vi "My_DHT11_Labview1_Gweb.vi"() -> ()   [LabVIEW 2024]
uses:
  <vilib>/Instr/_visa.llb/VISA Configure Serial Port (Instr).vi
  GlobalHum1.vi
  GlobalFan2.vi
  GlobalTemp1.vi
  GlobalFan1.vi
panel:
  in  "Tab Control 2":enum32{"Hum Chart", "Hum Gauge"}(tab)
  out "Waveform Chart 2":dbl(graph)
  out "Gauge 2":dbl(knob) scale=0.0..100.0 scale format="%%%#_g"
  in  "Tab Control":enum32{"Temp Chart", "Temp Gauge"}(tab)
  out "Waveform Chart":dbl(graph)
  out "Gauge":dbl(knob) scale=0.0..50.0
  out "Fan LED 2":bool
  out "Fan LED":bool
  in  "Fan":bool
  out "Humidity":dbl(slide) scale=0.0..100.0 scale format="%%%d"
  out "Temperature":dbl(slide) scale=0.0..100.0
  in  "?":bool
  in  "VISA Arduino Uno":refnum<visa-resource-name>
  in  "Fan2":bool
  # "Environmental Control System for Greenhouses\n\nMonitoring System"
  # "House No. 1"
  # "C"
  # "%"
  # "Eng. Yahia Gaddal\ngaddal18@gmail.com"
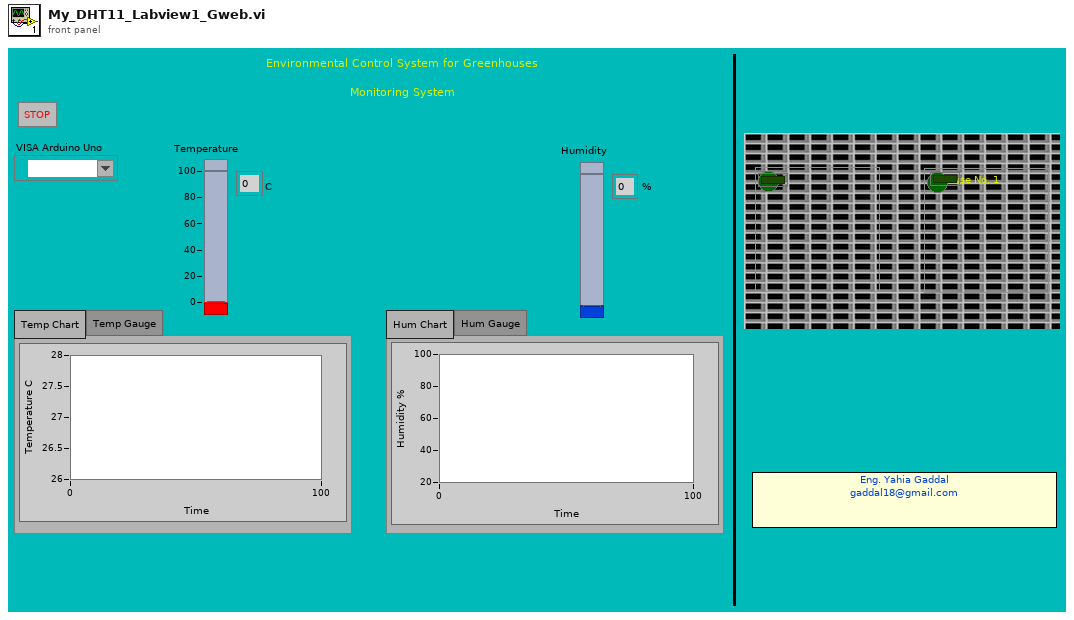
[diagram p1: front panel]
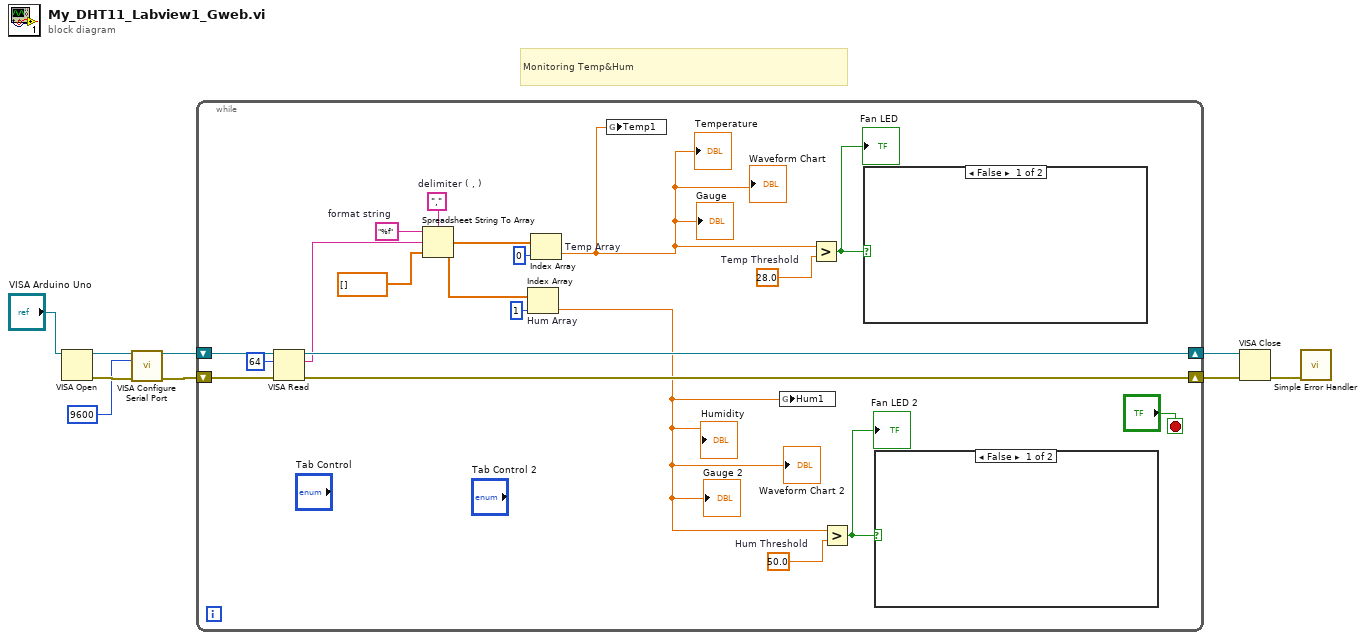
[diagram p0: block diagram]
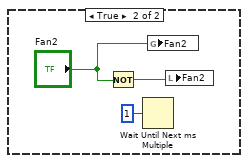
[diagram p2: hidden frame]
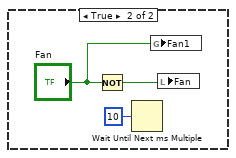
[diagram p3: hidden frame]
diagram:
  # "Monitoring Temp&Hum"
  n1 = VISA Open(VISA resource name="VISA Arduino Uno") -> (VISA resource name=w9:refnum<visa-resource-name>, error out=w8:errorcluster)  [unwired: 4 in]
  n2 = call-poly "VISA Configure Serial Port"("VISA resource name"=w9, "baud rate (9600)"=u32 9600, "error in (no error)"=w8) -> ("VISA resource name out"=w7:refnum<visa-resource-name>, "error out"=w6:errorcluster)  [unwired: 11 in]
  n3 = while {
    shift-right: [w26] -> w5
    shift-left: w7 -> [w28]
    shift-right: [w25] -> w4
    shift-left: w6 -> [w27]
    stop <- "?" stop-if-true
    w14 = 50.0  # Hum Threshold
    w18 = ","  # delimiter ( , )
    w21 = "%f"  # format string
    w23 = 28.0  # Temp Threshold
    n4 = VISA Read(VISA resource name=w28, byte count=u32 64, error in (no error)=w27) -> (VISA resource name out=w26:refnum<visa-resource-name>, read buffer=w20:string, error out=w25:errorcluster)  [unwired: 1 out]
    n5 = Spreadsheet String To Array(delimiter (Tab)=w18, format string=w21, spreadsheet string=w20, array type (2D Dbl)=dbl[] []) -> (array=w16:dbl[])
    n6 = Index Array "Hum Array"(array=w16, index=1) -> (element=w10:dbl)
    "Humidity" <- w10
    "Waveform Chart 2" <- w10
    "Gauge 2" <- w10
    n7 = Index Array "Temp Array"(array=w16, index=0) -> (element=w11:dbl)
    "Temperature" <- w11
    "Gauge" <- w11
    "Waveform Chart" <- w11
    n8 = global write "GlobalTemp1.vi" "Temp1"(w11) -> ()
    n9 = global write "GlobalHum1.vi" "Hum1"(w10) -> ()
    n10 = Greater?(x=w11, y=w23) -> (0:w22:bool)
    "Fan LED" <- w22
    n11 = Greater?(x=w10, y=w14) -> (0:w13:bool)
    "Fan LED 2" <- w13
    n12 = case shown="False" w22 {
      frame False {
      }
      frame True {
        n13 = Not(x="Fan") -> (.not. x?=w33:bool)
        n14 = Wait Until Next ms Multiple(millisecond multiple=u32 10) -> ()  [unwired: 1 out]
        n15 = global write "GlobalFan1.vi" "Fan1"("Fan") -> ()
        n16 = local write "Fan"(w33) -> ()
      }
    }
    n17 = case shown="False" w13 {
      frame False {
      }
      frame True {
        n18 = Not(x="Fan2") -> (.not. x?=w29:bool)
        n19 = Wait Until Next ms Multiple(millisecond multiple=u32 1) -> ()  [unwired: 1 out]
        n20 = global write "GlobalFan2.vi" "Fan2"("Fan2") -> ()
        n21 = local write "Fan2"(w29) -> ()
      }
    }
  }
  n22 = VISA Close(VISA resource name=w5, error in (no error)=w4) -> (error out=w1:errorcluster)
  n23 = call <vilib>:"Simple Error Handler.vi"("error in (no error)"=w1) -> ()  [unwired: 4 in, 5 out]
